vi "PH_Beckhoff_PP_PU.evt Call PSU set Voltage.vi"(0 "i ref in":refnum<vi>, 2 "PU":T1, 4 "Voltage to set [V]":dbl, 5 "error in":errorcluster, 6 "Limits [V]":cluster{"Lower":dbl, "Upper":dbl}) -> (14 "i ref out":refnum<vi>, 19 "error out":errorcluster)   [LabVIEW 2014, in "PH_Beckhoff_PP_PU.lvlib"]
doc: "This VI calls an event by a simple call."
uses:
  PH_Beckhoff_PP_PU.lvlib
  PH_PP_Common/PH_PP_Common.PUs.ctl
  PH_PP_Common/PH_PP_Common.PSU Tags.ctl
  PH_Beckhoff/PH_Beckhoff.lvlib
  PH_PP_Common/PH_PP_Common.lvlib
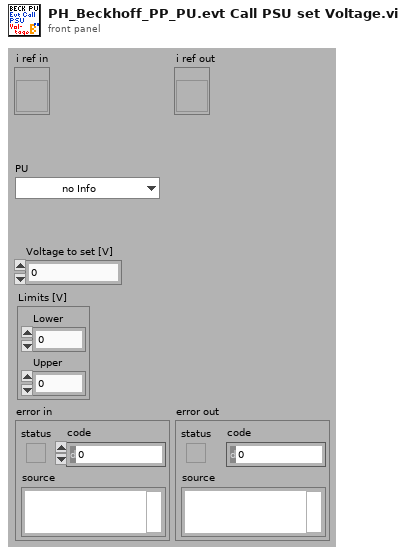
[diagram p1: front panel]
types:
  T1 = typedef "PH_PP_Common.lvlib/PH_PP_Common.PUs.ctl" = enum16{"no Info", "PA-19mm-1", "PA-19mm-2", "PA-45mm-PILC", "PA-45mm-MAIN", "MA-PU-1", "MA-PU-2", "MA-PU-3", "MA-PU-4", "MA-PU-5", "MA-PU-6", "MA-FR", "MA-PILC", "PA-45mm-DP"}
  T2 = typedef "PH_PP_Common.lvlib/PH_PP_Common.PSU Tags.ctl" = enum16{"voltage-indicator", "peak-detect", "current", "voltage", "inihibit-indicator", "end-of-charge", "HV-on-indicator", "overtemperature", "interlock-indicator", "load-fault", "sum-fault", "HV-off-indicator", "DC-ok", "inhibit", "HV-on", "interlock", "reset", "Status", "Limits"}
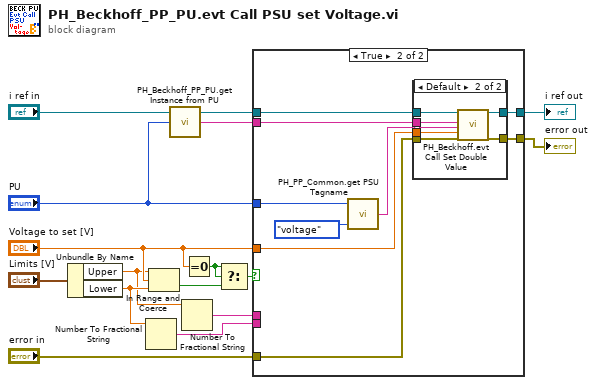
[diagram p0: block diagram]
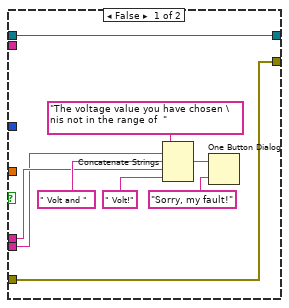
[diagram p2: hidden frame]
diagram:
  n1 = Unbundle By Name("Limits [V]") -> ("Upper"=w3:dbl, "Lower"=w5:dbl)
  n2 = Number To Fractional String(number=w5) -> (F-format string=w4:string)  [unwired: 3 in]
  n3 = In Range and Coerce(upper limit=w3, x="Voltage to set [V]", lower limit=w5) -> (In Range?=w9:bool)  [unwired: 1 out]
  n4 = call "PH_Beckhoff_PP_PU.get Instance from PU.vi"("PU"="PU") -> ("Beckhoff PU Instance"=w2:string)
  n5 = Number To Fractional String(number=w3) -> (F-format string=w6:string)  [unwired: 3 in]
  n6 = Equal To 0?(x="Voltage to set [V]") -> (x = 0?=w10:bool)
  n7 = Select(t=w10, s=w10, f=w9) -> (s? t:f=w8:bool)
  n8 = case shown="True" w8 {
    tunnel: "PU" -> [_ w33]
    tunnel: [w23 w32] -> w15
    tunnel: w2 -> [_ w31]
    tunnel: "error in" -> [w23 w30]
    tunnel: [w24 w29] -> w13
    tunnel: "i ref in" -> [w24 w28]
    tunnel: "Voltage to set [V]" -> [_ w25]
    tunnel: w6 -> [w17 _]
    tunnel: w4 -> [w16 _]
    frame False {
      n9 = Concatenate Strings("The voltage value you have chosen \nis not in the range of  ", w16, " Volt and ", w17, " Volt!") -> (w22:string)
      n10 = One Button Dialog(message=w22, button name ("OK")="Sorry, my fault!") -> ()  [unwired: 1 out]
    }
    frame True {
      n11 = call "PH_PP_Common.get PSU Tagname.vi"("PSU Tag"=PH_PP_Common.PSU_Tags."voltage", "PU"=w33) -> ("PSU Tagname"=w27:string)  [unwired: 1 in]
      n12 = case shown="Default" w27 {
        selector: w27 -> [_ w37]
        tunnel: [w34 w42] -> w32
        tunnel: w31 -> [_ w41]
        tunnel: w30 -> [w34 w40]
        tunnel: [w35 w39] -> w29
        tunnel: w28 -> [w35 w38]
        tunnel: w25 -> [_ w36]
        frame "", "N/A" {
        }
        frame Default {
          n13 = call "PH_Beckhoff.evt Call Set Double Value.vi"("i ref in"=w38, "Beckhoff Instance"=w41, "Tagname to set"=w37, "Value"=w36, "error in"=w40) -> ("i ref out"=w39:refnum<vi>, "error out"=w42:errorcluster)  [unwired: 13 in]
        }
      }
    }
  }
  "error out" <- w15
  "i ref out" <- w13
